vi "example_03_json_convert.vi"() -> ()   [LabVIEW 2015, in "lv-unit-conversion.lvlib"]
uses:
  lv-unit-conversion.lvlib
  public/advanced/load_dictionary_json.vi
panel:
  out "time_to_read":dbl format="%<%H:%M:%S%3u>t"
  out "value out":dbl
  in  "value in":dbl
  in  "source_unit":string="m"
  in  "conversion_unit":string="in"
  out "unit_dictionary":variant
  out "error out":errorcluster
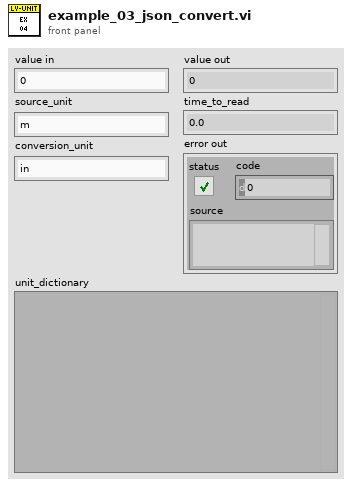
[diagram p1: front panel]
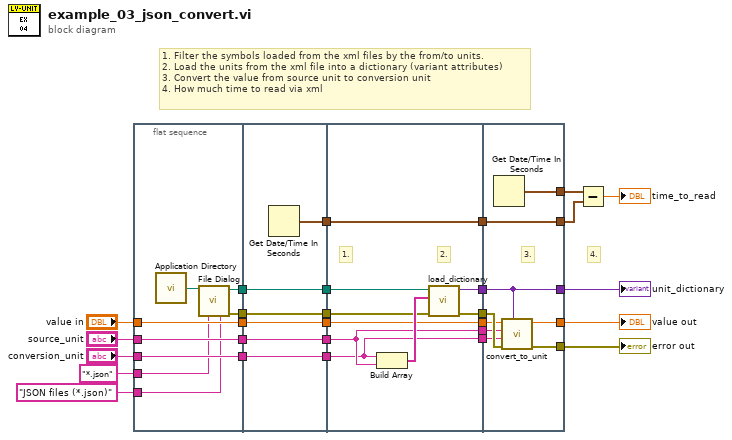
[diagram p0: block diagram]
diagram:
  # "4."
  # "1. Filter the symbols loaded from the xml files by the from/to units.\n2. Load the units from the xml file into a dictionary (variant attributes)\n3. Convert the value from source unit to conversion unit\n4. How much time to read via xml"
  n1 = flat-sequence {
    tunnel: "value in" -> [w34]
    tunnel: "conversion_unit" -> [w35]
    tunnel: "source_unit" -> [w36]
    tunnel: [w36] -> w28
    tunnel: [w35] -> w27
    tunnel: [w34] -> w26
    tunnel: [w33] -> w25
    tunnel: [w32] -> w24
    tunnel: "*.json" ("pattern (all files)") -> [w31]
    tunnel: "JSON files (*.json)" ("pattern label") -> [w30]
    tunnel: w28 -> [w42]
    tunnel: [w42] -> w23
    tunnel: w27 -> [w41]
    tunnel: [w41] -> w22
    tunnel: w26 -> [w40]
    tunnel: [w40] -> w21
    tunnel: [w37] -> w20
    tunnel: w25 -> [w39]
    tunnel: [w39] -> w19
    tunnel: w24 -> [w38]
    tunnel: [w38] -> w18
    tunnel: [w51] -> w17
    tunnel: [w50] -> w16
    tunnel: [w48] -> w15
    tunnel: [w47] -> w14
    tunnel: [w46] -> w13
    tunnel: [w45] -> w12
    tunnel: w23 -> [w47]
    tunnel: w22 -> [w46]
    tunnel: w21 -> [w48]
    tunnel: w20 -> [w45]
    tunnel: w19 -> [w44]
    tunnel: w18 -> [w43]
    tunnel: [w59] -> w9
    tunnel: w17 -> [w60]
    tunnel: w16 -> [w59]
    tunnel: w15 -> [w58]
    tunnel: w14 -> [w57]
    tunnel: w13 -> [w56]
    tunnel: [w55] -> w7
    tunnel: [w54] -> w6
    tunnel: w12 -> [w53]
    tunnel: [w53] -> w4
    tunnel: [w52] -> w5
    frame #0 {
      n2 = call <vilib>:"Application Directory.vi"() -> ("Application Directory"=w29:path)
      n3 = call "File Dialog"("start path"=w29, "pattern (all files)"=w31, "pattern label"=w30) -> ("selected path"=w32:path, "error out"=w33:errorcluster)  [unwired: 9 in, 2 out]
    }
    frame #1 {
      n4 = Get Date/Time In Seconds() -> (seconds since 1Jan1904=w37:timestamp)
    }
    frame #2 {
      # "2."
      # "1."
      n5 = Build Array(w46, w47) -> (w49:string[])
      n6 = call-poly "load_dictionary.vi"("error in (no error)"=w44, "symbols []"=w49, "json_path"=w43) -> ("error out"=w51:errorcluster, "unit_dictionary"=w50:variant)  [unwired: 7 in]
    }
    frame #3 {
      # "3."
      n7 = Get Date/Time In Seconds() -> (seconds since 1Jan1904=w52:timestamp)
      n8 = call "convert_to_unit.vi"("unit_dictionary"=w59, "error in (no error)"=w60, "unit_to"=w56, "unit_from"=w57, "value in"=w58) -> ("error out"=w54:errorcluster, "value out"=w55:dbl)  [unwired: 5 in]
    }
  }
  n9 = Subtract(x=w5, y=w4) -> (x-y=→"time_to_read":dbl)
  "error out" <- w6
  "unit_dictionary" <- w9
  "value out" <- w7
